vi "Configure Measurement.vi"(0 "VISA resource name":refnum<visa-resource-name>, 1 "Corrected Power Standard (0: IEC76-1(1976))":i32(ring) items=["IEC76-1(1976)", "IEC76-1(1993)"], 2 "Power Equation Type (0: Type1)":i32(ring) items=["Type1", "Type2", "Type3"], 3 "Apparent Power Equation (0: Urms * Irms)":i32(ring) items=["Urms * Irms", "Umean * Imean", "Udc * Idc", "Umean * Irms", "Urmean * Irmean"], 5 "Corrected Power Coefficients 1 (0.5000)":dbl=0.5 min=0.0001 max=9.9999 format="%.4f", 7 "Corrected Power Coefficients 2 (0.5000)":dbl=0.5 min=0.0001 max=9.9999 format="%.4f", 9 "Sampling Frequency (0: Auto)":i32(ring) items=["Auto", "2.000000MHz", "1.941176MHz", "1.885714MHz"], 11 "error in (no error)":errorcluster, 12 "Phase Difference Format (180 degrees)":i32(ring)=180 items=["180"=180, "360"=360], 13 "Synchronized Measurement (0: Master)":i32(ring) items=["Master", "Slave"]) -> (4 "VISA resource name out":refnum<visa-resource-name>, 15 "error out":errorcluster)   [LabVIEW 2021, in "Yokogawa WT1800 Series.lvlib"]
doc: "Configures the measurement features."
uses:
  <instrlib>/Yokogawa WT1800 Series/Yokogawa WT1800 Series.lvlib
panel:
  # "degrees"
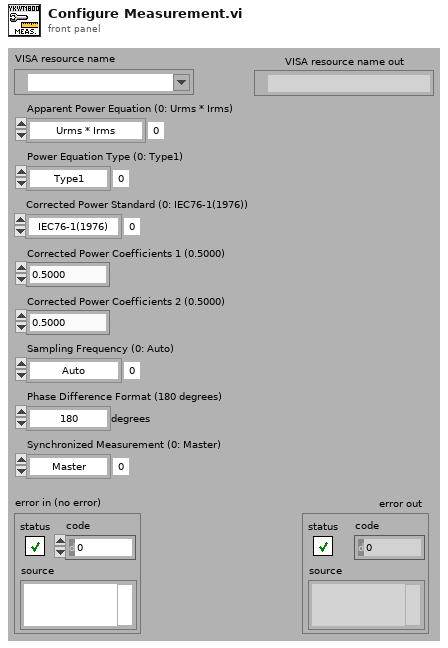
[diagram p1: front panel]
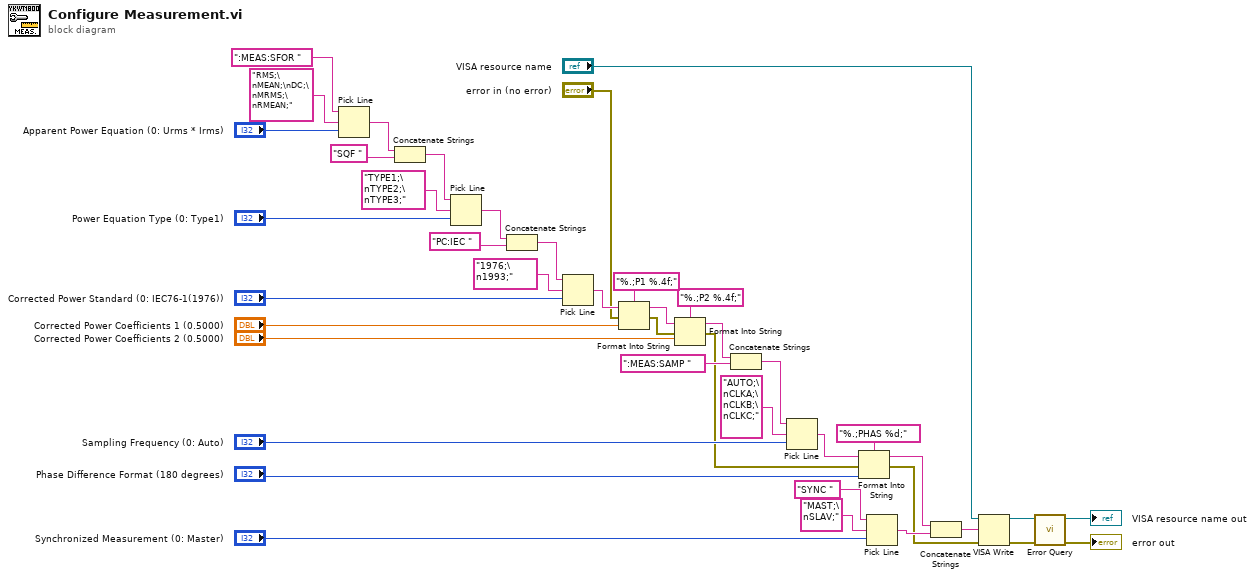
[diagram p0: block diagram]
diagram:
  n1 = Pick Line ("ライン選択")(string ("")=":MEAS:SFOR ", multi-line string="RMS;\nMEAN;\nDC;\nMRMS;\nRMEAN;" ("複数行文字列"), line index="Apparent Power Equation (0: Urms * Irms)") -> (output string=w19:string)
  n2 = Concatenate Strings(w19, "SQF ") -> (w21:string)
  n3 = Pick Line ("ライン選択")(string ("")=w21, multi-line string="TYPE1;\nTYPE2;\nTYPE3;" ("複数行文字列"), line index="Power Equation Type (0: Type1)") -> (output string=w1:string)
  n4 = Concatenate Strings(w1, "PC:IEC ") -> (w17:string)
  n5 = Pick Line ("ライン選択")(string ("")=w17, multi-line string="1976;\n1993;" ("複数行文字列"), line index="Corrected Power Standard (0: IEC76-1(1976))") -> (output string=w13:string)
  n6 = Format Into String(format string="%.;P1 %.4f;" ("形式文字列"), initial string=w13, error in="error in (no error)", "Corrected Power Coefficients 1 (0.5000)") -> (resulting string=w8:string, error out=w7:errorcluster)
  n7 = Format Into String(format string="%.;P2 %.4f;" ("形式文字列"), initial string=w8, error in=w7, "Corrected Power Coefficients 2 (0.5000)") -> (resulting string=w4:string, error out=w2:errorcluster)
  n8 = Concatenate Strings(w4, ":MEAS:SAMP ") -> (w3:string)
  n9 = Pick Line ("ライン選択")(string ("")=w3, multi-line string="AUTO;\nCLKA;\nCLKB;\nCLKC;" ("複数行文字列"), line index="Sampling Frequency (0: Auto)") -> (output string=w35:string)
  n10 = Format Into String(format string="%.;PHAS %d;" ("形式文字列"), initial string=w35, error in=w2, "Phase Difference Format (180 degrees)") -> (resulting string=w30:string, error out=w29:errorcluster)
  n11 = Pick Line ("ライン選択")(string ("")="SYNC ", multi-line string="MAST;\nSLAV;" ("複数行文字列"), line index="Synchronized Measurement (0: Master)") -> (output string=w31:string)
  n12 = Concatenate Strings(w30, w31) -> (w28:string)
  n13 = VISA Write ("VISA書き込み")(VISA resource name="VISA resource name", write buffer=w28, error in (no error)=w29) -> (VISA resource name out=w42:refnum<visa-resource-name>, error out=w41:errorcluster)  [unwired: 1 out]
  n14 = call <instrlib>:"Error Query.vi"("error in (no error)"=w41, "VISA resource name"=w42) -> ("error out"=→"error out":errorcluster, "VISA resource name out"=→"VISA resource name out":refnum<visa-resource-name>)  [unwired: 6 in, 2 out]
